vi "main.vi"() -> ()   [LabVIEW 2024]
uses:
  states.ctl
panel:
  out "Czas":dbl
  out "Logi":string
  in  "LOGUJ":bool
  in  "EXIT":bool
  out "LED":bool
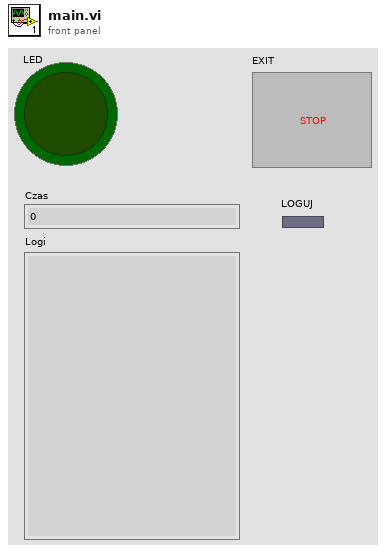
[diagram p1: front panel]
types:
  T1 = typedef "states.ctl" = enum16{"IDLE", "INIT", "LOG", "MOUSE", "EXIT"}
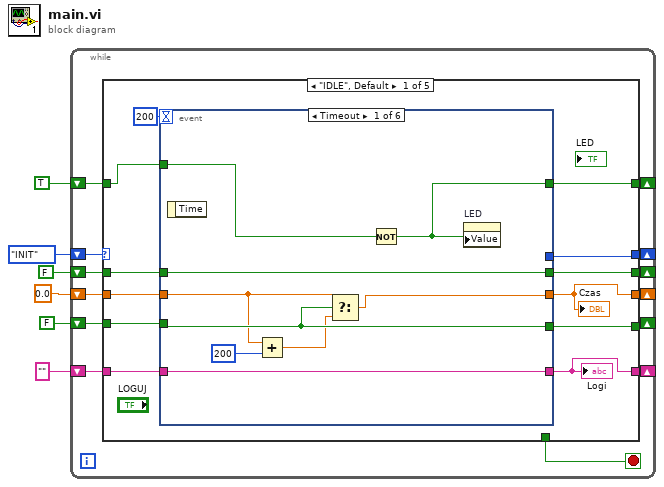
[diagram p0: block diagram]
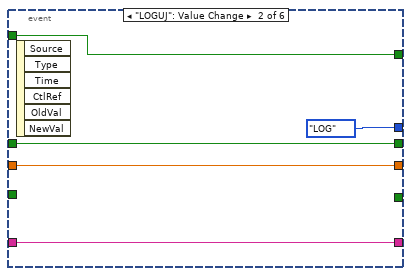
[diagram p2: hidden frame]
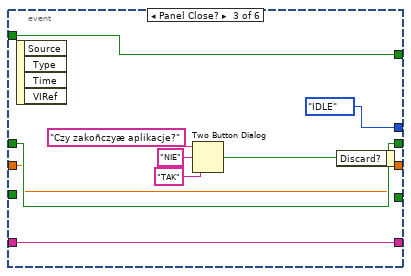
[diagram p3: hidden frame]
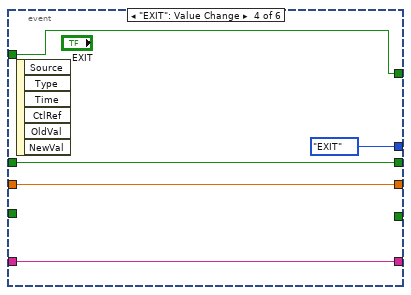
[diagram p4: hidden frame]
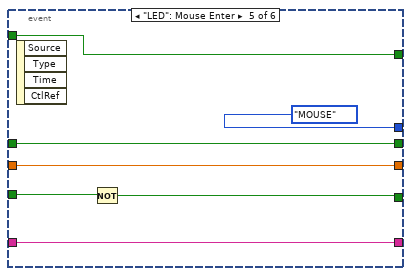
[diagram p5: hidden frame]
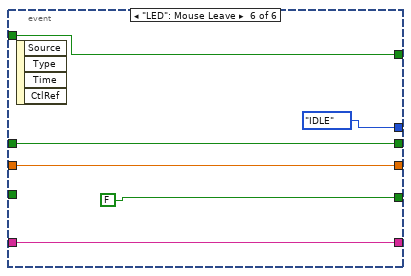
[diagram p6: hidden frame]
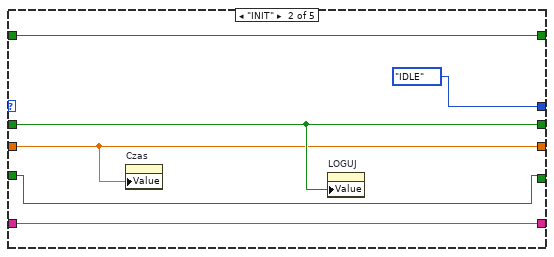
[diagram p7: hidden frame]
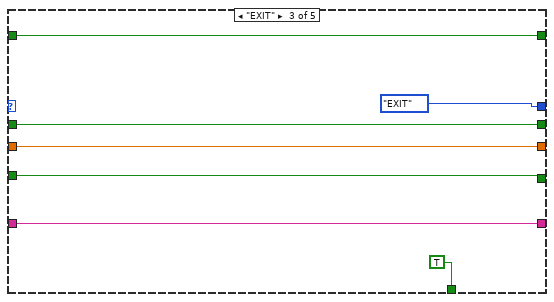
[diagram p8: hidden frame]
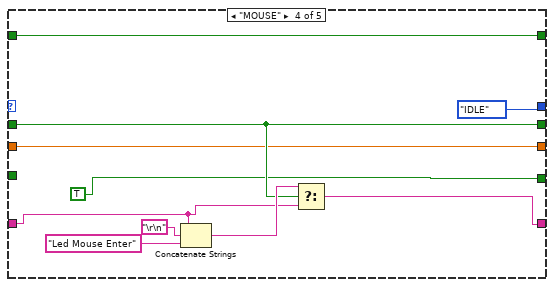
[diagram p9: hidden frame]
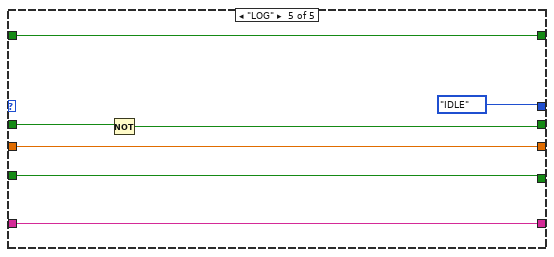
[diagram p10: hidden frame]
diagram:
  n1 = while {
    shift-right: [w16] -> _
    shift-left: states."INIT" -> [w19]
    shift-right: [w17] -> _
    shift-left: TRUE -> [w18]
    shift-right: [w12] -> _
    shift-left: "" -> [w14]
    shift-right: [w11] -> _
    shift-left: 0.0 -> [w13]
    shift-right: [w9] -> _
    shift-left: FALSE -> [w10]
    shift-right: [w7] -> _
    shift-left: FALSE -> [w8]
    stop <- w15 stop-if-true
    n2 = case shown="\"IDLE\", Default" w19 {
      tunnel: w18 -> [w30 w78 w83 w95 w102]
      tunnel: [w28 w78 w83 w95 w102] -> w17
      tunnel: [w29 states."IDLE" states."EXIT" states."IDLE" states."IDLE"] -> w16
      tunnel: [_ _ TRUE _ _] -> w15
      tunnel: w14 -> [w27 w77 w81 w89 w97]
      tunnel: w13 -> [w25 w74 w82 w87 w98]
      tunnel: [w26 w77 w81 w91 w97] -> w12
      tunnel: [w22 w74 w82 w87 w98] -> w11
      tunnel: w10 -> [w24 w76 w80 w88 w100]
      tunnel: [w23 w76 w80 w88 w99] -> w9
      tunnel: w8 -> [w21 w75 w79 _ w96]
      tunnel: [w20 w75 w79 TRUE w96] -> w7
      frame "IDLE", Default {
        n3 = event shown="[0] Timeout" {
          selector: _ -> [_ _ _ _ _ _]
          dyn-events: _ -> [_ _ _ _ _ _]
          timeout: 200 -> [_ _ _ _ _ _]
          tunnel: w30 -> [w40 w42 w48 w56 w63 w67]
          tunnel: [_ states."LOG" states."IDLE" states."EXIT" states."MOUSE" states."IDLE"] -> w29
          tunnel: [w39 w42 w48 w56 w63 w67] -> w28
          tunnel: w27 -> [w38 w43 w47 w57 w64 w72]
          tunnel: [w38 w43 w47 w57 w64 w72] -> w26
          tunnel: w25 -> [w34 w44 w49 w58 w65 w70]
          tunnel: [w35 w44 w49 w58 w65 w70] -> w22
          tunnel: w24 -> [w37 w41 w50 w55 w62 w69]
          tunnel: [w37 w41 w50 w55 w62 w69] -> w23
          tunnel: w21 -> [w36 _ _ _ w61 _]
          tunnel: [w36 _ _ _ w60 FALSE] -> w20
          event Timeout {
            n4 = event-data() -> ()  [unwired: 1 in, 1 out]
            n5 = Add(x=w34, y=200) -> (x+y=w33:dbl)
            n6 = Select(t=w34, s=w36, f=w33) -> (s? t:f=w35:dbl)
            n7 = Not(x=w40) -> (.not. x?=w39:bool)
            n8 = property on="LED" class="Bool (strict)"("Value"=w39) -> ()  [unwired: 2 in, 2 out]
          }
          event "LOGUJ": Value Change {
            n9 = event-data() -> ()  [unwired: 1 in, 6 out]
          }
          event Panel Close? {
            n10 = event-data() -> ()  [unwired: 1 in, 4 out]
            n11 = Two Button Dialog(message="Czy zakoñczyæ aplikacje?", 1:"TAK" ("F button name (\"Cancel\")"), 2:"NIE" ("T button name (\"OK\")")) -> (T button?=w46:bool)
            n12 = event-data("Discard?"=w46) -> ()  [unwired: 1 in, 1 out]
          }
          event "EXIT": Value Change {
            n13 = event-data() -> ()  [unwired: 1 in, 6 out]
          }
          event "LED": Mouse Enter {
            n14 = event-data() -> ()  [unwired: 1 in, 4 out]
            n15 = Not(x=w61) -> (.not. x?=w60:bool)
          }
          event "LED": Mouse Leave {
            n16 = event-data() -> ()  [unwired: 1 in, 4 out]
          }
        }
        "Logi" <- w26
        "Czas" <- w22
      }
      frame "INIT" {
        n17 = property on="Czas" class="DigNum (strict)"("Value"=w74) -> ()  [unwired: 2 in, 2 out]
        n18 = property on="LOGUJ" class="Bool (strict)"("Value"=w76) -> ()  [unwired: 2 in, 2 out]
      }
      frame "EXIT" {
      }
      frame "MOUSE" {
        n19 = Concatenate Strings(w89, "\r\n", "Led Mouse Enter") -> (w90:string)
        n20 = Select(t=w90, s=w88, f=w89) -> (s? t:f=w91:string)
      }
      frame "LOG" {
        n21 = Not(x=w100) -> (.not. x?=w99:bool)
      }
    }
  }
